vi "Calibration.vi"() -> ()   [LabVIEW 2009]
uses:
  lib/Calibration/Actuator Controls.ctl
  lib/Apps/On Off Button.ctl
  lib/Calibration/Calibration Readings.ctl
  lib/Calibration/CalibrationRampState.ctl
  lib/Calibration/SquareWaveRampState.ctl
  lib/Data Access Objects/Autobalance/Autobalance Control Parameters.ctl
  lib/Calibration/Cal Autobalance State.ctl
  lib/Apps/Yes No Button.ctl
  lib/Autobalance/Autobalance Stage.ctl
  lib/Calibration/Cal Autobalance Loop States.ctl
  lib/Autobalance/Autobalance State.ctl
  Test Utilities/DAQ Read Actions.ctl
  <vilib>/DAQmx/write.llb/DAQmx Write (Analog 1D DBL NChan 1Samp).vi
  lib/Autobalance/Autobalance Status Data.ctl
  lib/Autobalance/Autobalance Data Point.ctl
  lib/Data Access Objects/Metadata/LBCB Number.ctl
panel:
  in  "Control Type":enum32{"Set", "Ramp", "Square", "Autobalance"}(tab)=enum."Autobalance"
  in  "Set Control":cluster{"Set":bool, "Actuator Controls":T1} {"Actuator Controls"."Actuator Z2" min=-10.0 max=10.0 step=0.1 scale=-10.0..10.0; "Actuator Controls"."Actuator Z3" min=-10.0 max=10.0 step=0.1 scale=-10.0..10.0; "Actuator Controls"."Actuator X2" min=-10.0 max=10.0 step=0.1 scale=-10.0..10.0; "Actuator Controls"."Actuator Y1" min=-10.0 max=10.0 step=0.1 scale=-10.0..10.0; "Actuator Controls"."Actuator Z1" min=-10.0 max=10.0 step=0.1 scale=-10.0..10.0; "Actuator Controls"."Actuator X1" min=-10.0 max=10.0 step=0.1 scale=-10.0..10.0}
  in  "Ramp Control":T2={"Ramp Time\n(millseconds)"=30.0, "No. of Steps"=100, "Ramp"=FALSE, "Actuator Controls"={"Actuator X1"=0.0, "Actuator X2"=0.0, "Actuator Y1"=0.0, "Actuator Z1"=0.0, "Actuator Z2"=0.0, "Actuator Z3"=0.0}} {"Actuator Controls"."Actuator Z2" min=-10.0 max=10.0 step=0.1 scale=-10.0..10.0; "Actuator Controls"."Actuator Z3" min=-10.0 max=10.0 step=0.1 scale=-10.0..10.0; "Actuator Controls"."Actuator X2" min=-10.0 max=10.0 step=0.1 scale=-10.0..10.0; "Actuator Controls"."Actuator Y1" min=-10.0 max=10.0 step=0.1 scale=-10.0..10.0; "Actuator Controls"."Actuator Z1" min=-10.0 max=10.0 step=0.1 scale=-10.0..10.0; "Actuator Controls"."Actuator X1" min=-10.0 max=10.0 step=0.1 scale=-10.0..10.0}
  in  "Ramp State":T3
  in  "Square State":T4
  in  "Square Control":T5={"Hold Time\n(milliseconds)"=2000, "No. of\n Iterations"=5, "Run"=FALSE, "Actuator Controls"={"Actuator X1"=0.0, "Actuator X2"=0.0, "Actuator Y1"=0.0, "Actuator Z1"=0.0, "Actuator Z2"=0.0, "Actuator Z3"=0.0}} {"Actuator Controls"."Actuator Z2" min=-10.0 max=10.0 step=0.1 scale=-10.0..10.0; "Actuator Controls"."Actuator Z3" min=-10.0 max=10.0 step=0.1 scale=-10.0..10.0; "Actuator Controls"."Actuator X2" min=-10.0 max=10.0 step=0.1 scale=-10.0..10.0; "Actuator Controls"."Actuator Y1" min=-10.0 max=10.0 step=0.1 scale=-10.0..10.0; "Actuator Controls"."Actuator Z1" min=-10.0 max=10.0 step=0.1 scale=-10.0..10.0; "Actuator Controls"."Actuator X1" min=-10.0 max=10.0 step=0.1 scale=-10.0..10.0}
  in  "Autobalance":bool
  in  "Error Tolerance":dbl=0.005
  out "Cal Autobalance State":T6
  in  "Autobalance \nControl Parameters":T9={"Number of Samples"=30, "Delay After Cmd"=100, "Maximum Command"=9.2}
  out "Autobalance Loop State":T10 caption="State"
  out "Autobalance State Out":T11
  in  "Zoom Type":T12(ring)
  in  "Restore":bool
  in  "Zoom In":bool
  in  "Readings":T13
  in  "Actuator":i32(listbox)
  out "Readings":T14(graph)={"Average[0]"=-7.17251209904047, "Average[1]"=-8.19396103384171, "Average[2]"=-9.68369051887908, "Average[3]"=-9.45574535938537, "Average[4]"=-9.241187346298316, "Average[5]"=-8.612741694704903, "Average[6]"=0.0, "Average[7]"=0.0, "Average[8]"=0.0}
  in  "Logging":T15
  out "Command Voltage":dbl[](array[numeric])=[-0.0, -0.0, -0.0, -0.0, -0.0, -0.0]
  in  "Log File Path":path=path "C:/Documents and Settings/mbletzin/Desktop/CalVolts.txt"
  out "Control Voltage":dbl[](array[numeric])=[-0.0, -0.0, -0.0, -0.0, -0.0, -0.0]
  in  "rate":dbl=100.0
  in  "samples per channel":i32=30
  out "Servo Error Reading":dbl[](array[numeric])=[-5.882376727117365, -6.585181568259441, -9.220694636240406, -8.950128810593748, -9.598174526274564, -9.458937013781334]
  in  "Command Voltage Task":refnum<k21>="Command Voltage"
  in  "Readings Task":refnum<k21>="All Readings"
  out "Read error out":errorcluster
  out "Write error out":errorcluster
  in  "Read error in (no error)":errorcluster
  out "Load Cell \nReading":dbl[](array[numeric])=[-7.680882880270997, -8.566659800159199, -9.658116593296763, -9.594949810916727, -8.940447035067507, -8.192445315897492]
  out "LVDT Reading":dbl[](array[numeric])=[-7.17251209904047, -8.19396103384171, -9.68369051887908, -9.45574535938537, -9.241187346298316, -8.612741694704903]
  in  "Quit":bool
  # "LBCB CALIBRATION PROGRAM"
  # "Is Balanced"
  # "State"
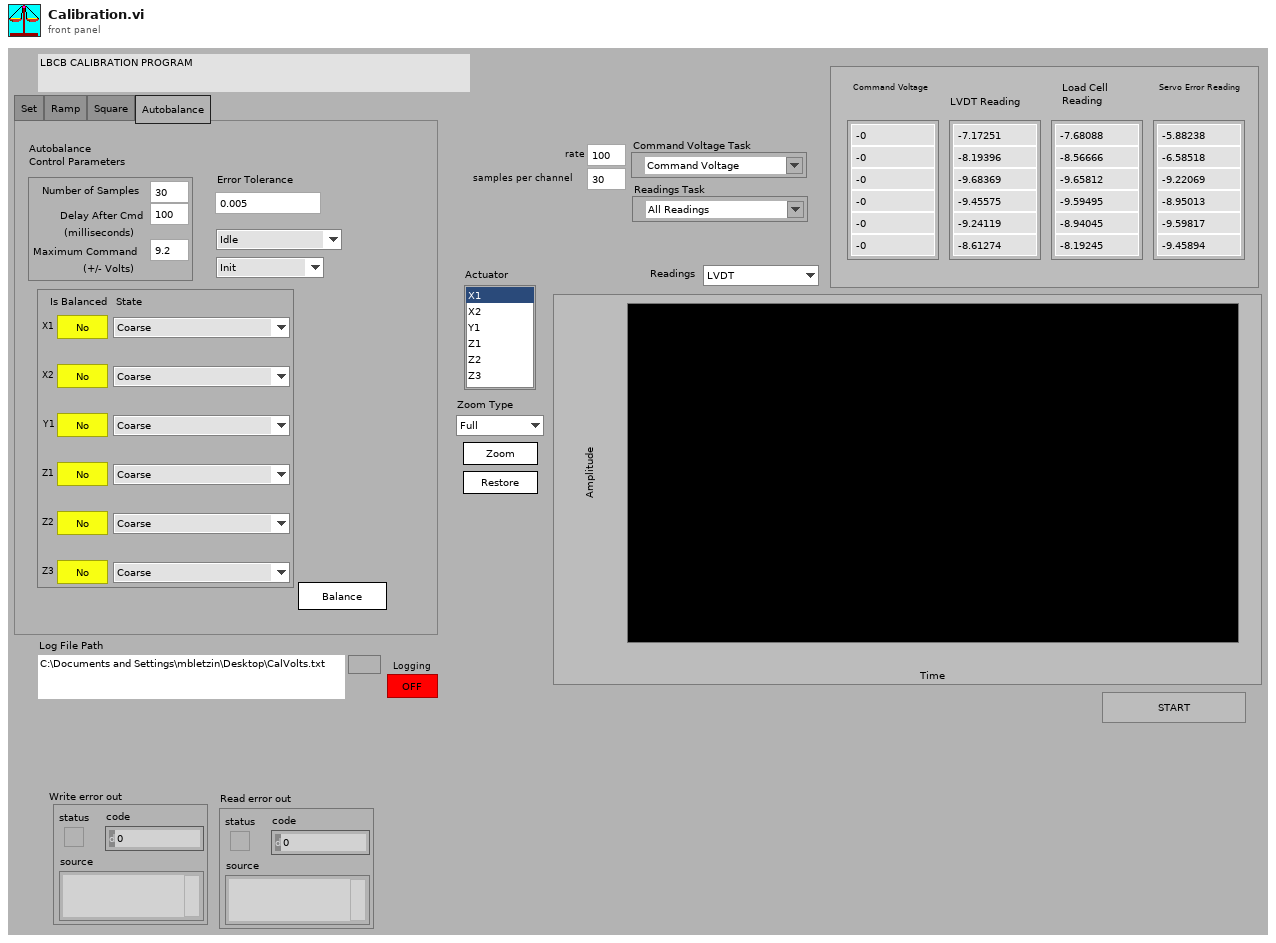
[diagram p1: front panel]
types:
  T1 = typedef "Actuator Controls.ctl" = cluster{"Actuator X1":dbl, "Actuator X2":dbl, "Actuator Y1":dbl, "Actuator Z1":dbl, "Actuator Z2":dbl, "Actuator Z3":dbl}
  T2 = cluster{"Ramp Time\n(millseconds)":dbl, "No. of Steps":i32, "Ramp":bool, "Actuator Controls":T1}
  T3 = typedef "CalibrationRampState.ctl" = enum16{"Idle", "Start Ramp", "Ramping", "Stopping"}
  T4 = typedef "SquareWaveRampState.ctl" = enum16{"Idle", "Start Wave", "High", "Low", "Stop"}
  T5 = cluster{"Hold Time\n(milliseconds)":i32, "No. of\n Iterations":i32, "Run":bool, "Actuator Controls":T1}
  T6 = typedef "Cal Autobalance State.ctl" = cluster{"X1 IsBalanced":T7, "X1 State":T8, "X2 IsBalanced":T7, "X2 State":T8, "Y1 IsBalanced":T7, "Y1 State":T8, "Z1 IsBalanced":T7, "Z1 State":T8, "Z2 IsBalanced":T7, "Z2 State":T8, "Z3 IsBalanced":T7, "Z3 State":T8}
  T7 = typedef "Yes No Button.ctl" = bool
  T8 = typedef "Autobalance Stage.ctl" = enum16{"Coarse", "Fine", "Backing Up", "Done"}
  T9 = typedef "Autobalance Control Parameters.ctl" = cluster{"Number of Samples":i32, "Delay After Cmd":i32, "Maximum Command":dbl}
  T10 = typedef "Cal Autobalance Loop States.ctl" = enum16{"Idle", "Start Balancing", "Balancing", "Stop"}
  T11 = typedef "Autobalance State.ctl" = enum16{"Init", "Send High ", "Wait High", "Read High Start", "Read High", "Send Low", "Wait Low", "Read Low Start", "Read Low", "Publish", "Calculate", "Done"}
  T12 = enum16{"Full", "Upper Half", "Upper Edge", "Lower Half", "Lower Edge"}
  T13 = typedef "Calibration Readings.ctl" = enum16{"LVDT", "Load Cell", "Servo Errors"}
  T14 = cluster{"Average[0]":dbl, "Average[1]":dbl, "Average[2]":dbl, "Average[3]":dbl, "Average[4]":dbl, "Average[5]":dbl, "Average[6]":dbl, "Average[7]":dbl, "Average[8]":dbl}
  T15 = typedef "On Off Button.ctl" = bool
  T16 = enum8{"Enabled", "Disabled", "Disabled and Grayed Out"}
  T17 = typedef "DAQ Read Actions.ctl" = enum16{"Start", "Read", "Stop"}
  T18 = typedef "Autobalance Status Data.ctl" = cluster{"IsBalanced":T7, "Autobalance Stage":T8, "High":T19, "Low":T19, "Balanced \nCmd":dbl}
  T19 = typedef "Autobalance Data Point.ctl" = cluster{"cCmd":dbl, "cServo":dbl, "pCmd":dbl, "pServo":dbl}
  T20 = typedef "LBCB Number.ctl" = enum16{"LBCB1", "LBCB2"}
  T21 = cluster{"Average[0]":dbl, "Average[1]":dbl, "Average[2]":dbl, "Average[3]":dbl, "Average[4]":dbl, "Average[5]":dbl, "Average[6]":dbl, "Average[7]":dbl, "Average[8]":dbl}[]
  T22 = enum16{"open", "replace", "create", "open or create", "replace or create", "replace or create with confirmation"}
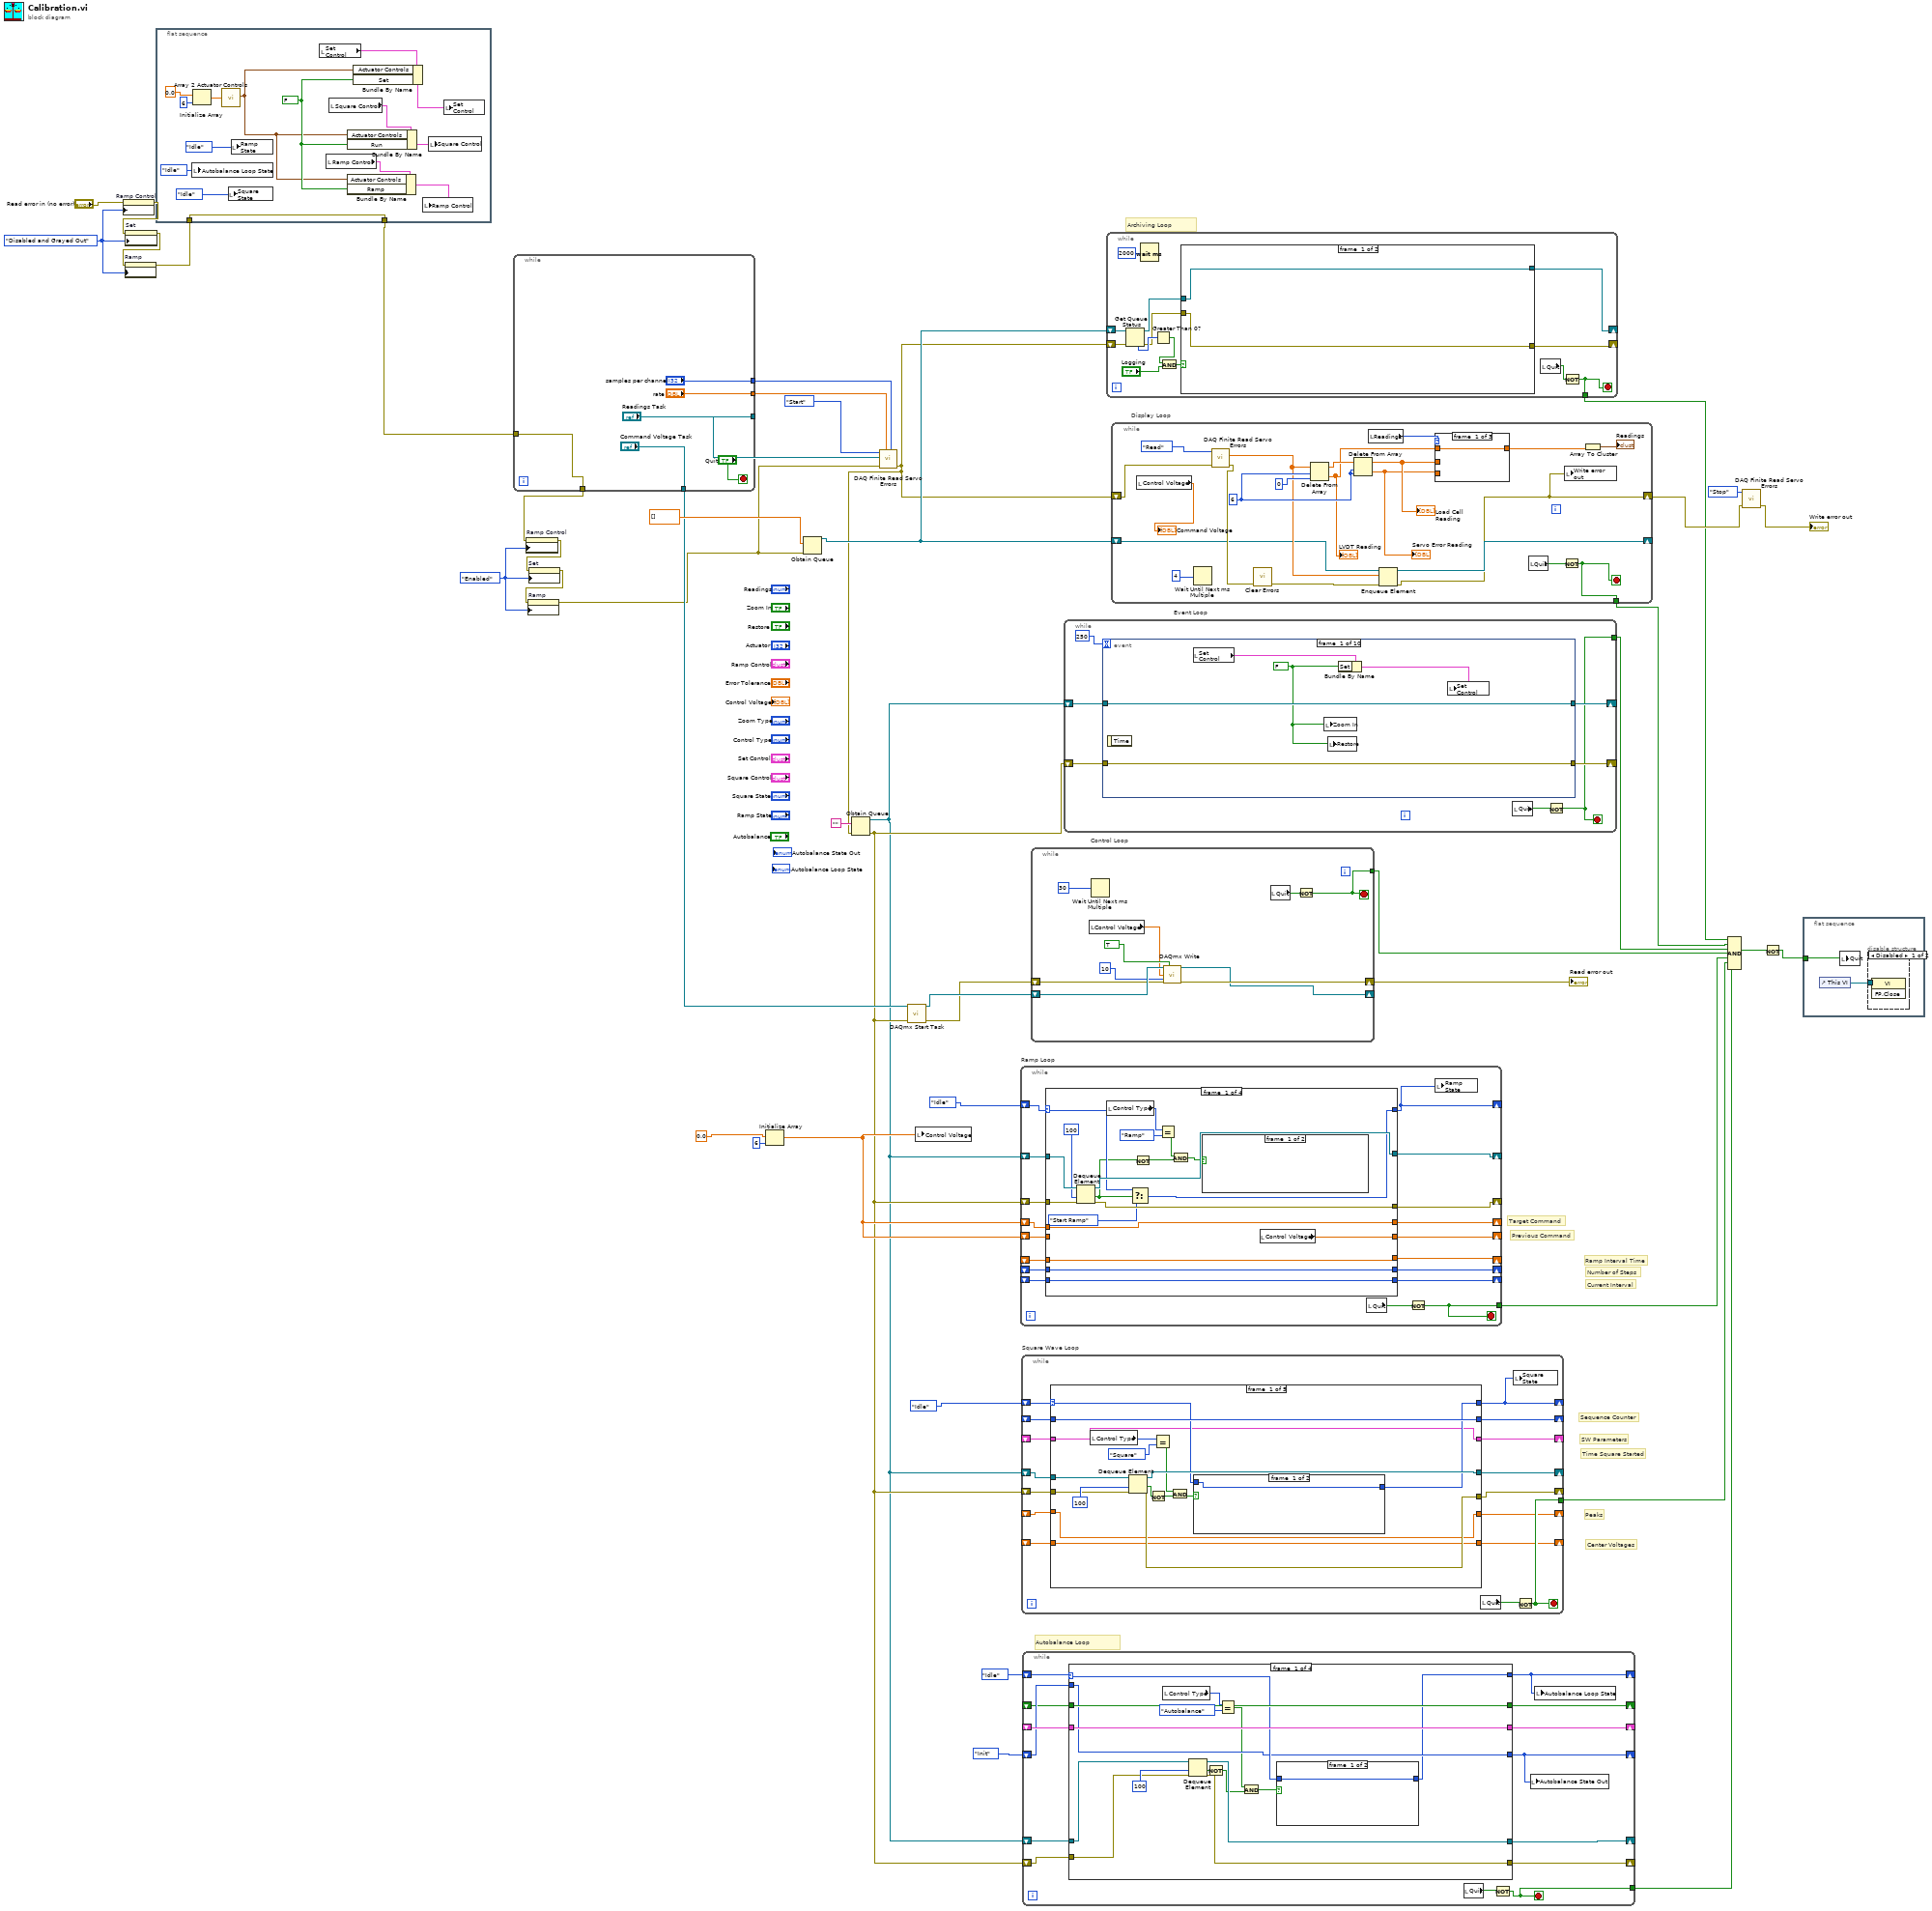
[diagram p0: block diagram]
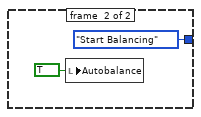
[diagram p2: hidden frame]
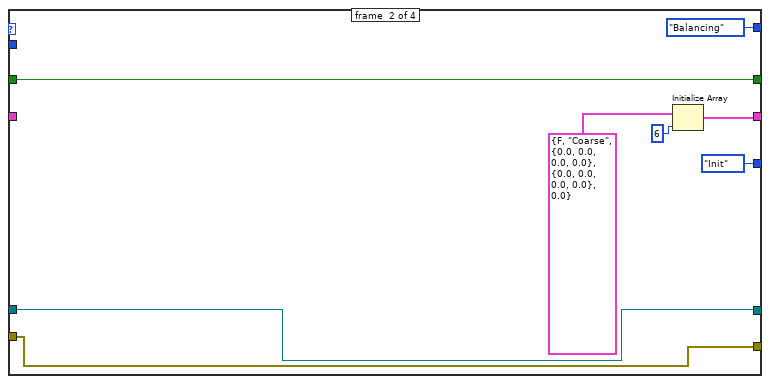
[diagram p3: hidden frame]
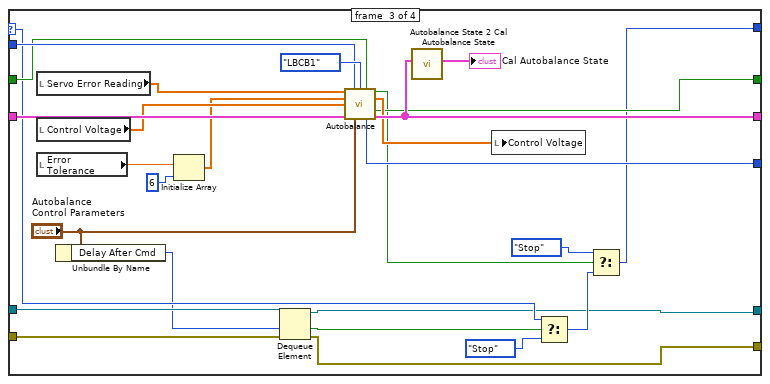
[diagram p4: hidden frame]
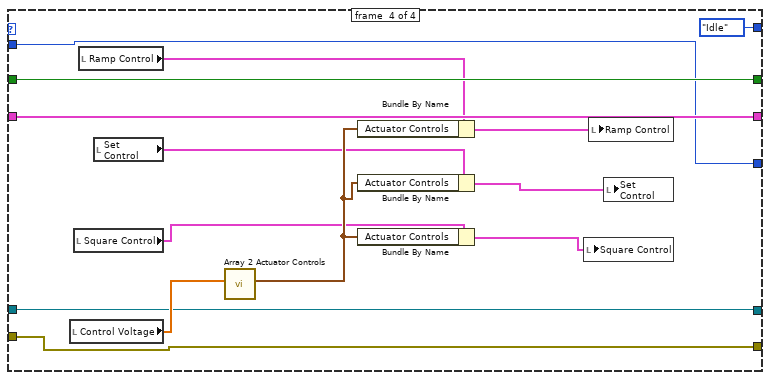
[diagram p5: hidden frame]
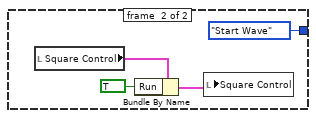
[diagram p6: hidden frame]
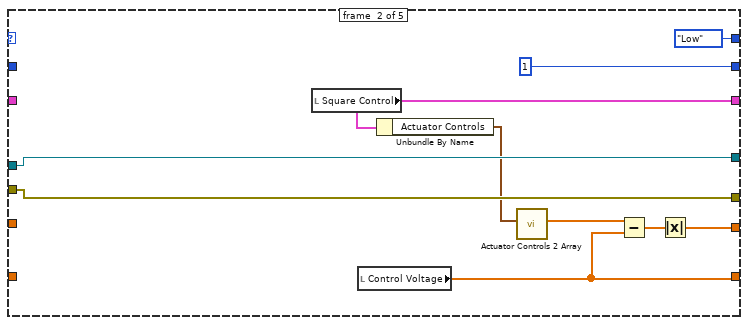
[diagram p7: hidden frame]
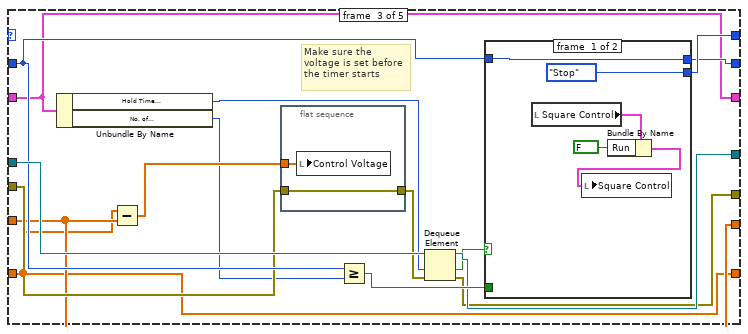
[diagram p8: hidden frame]
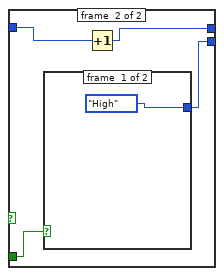
[diagram p9: hidden frame]
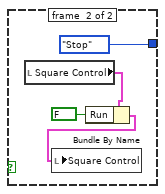
[diagram p10: hidden frame]
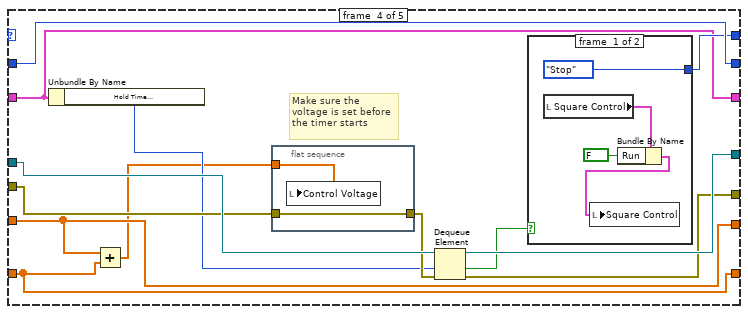
[diagram p11: hidden frame]
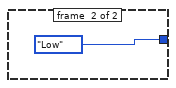
[diagram p12: hidden frame]
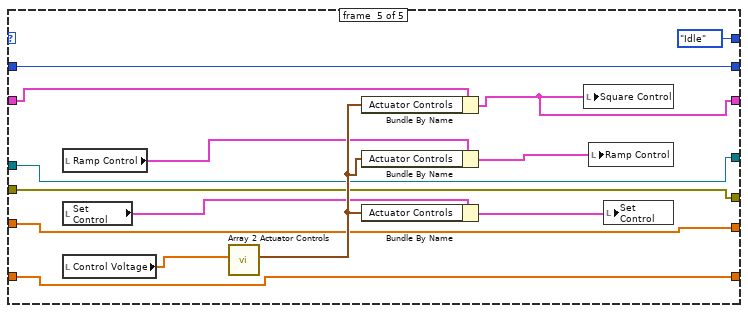
[diagram p13: hidden frame]
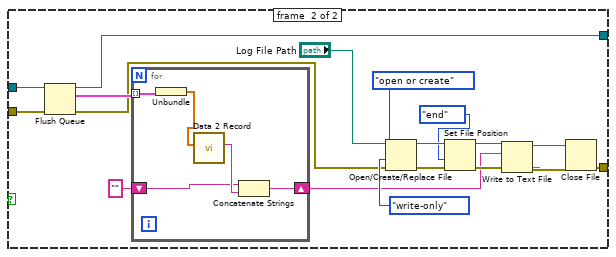
[diagram p15: hidden frame]
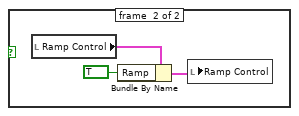
[diagram p16: hidden frame]
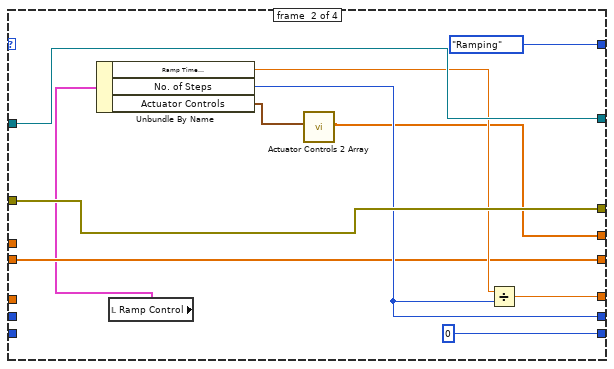
[diagram p17: hidden frame]
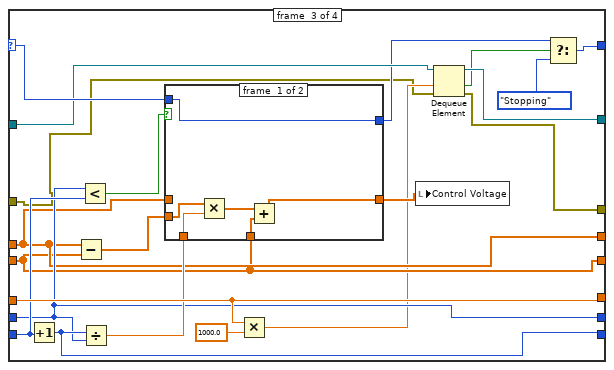
[diagram p18: hidden frame]
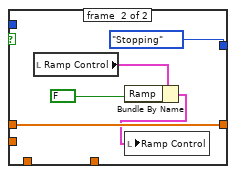
[diagram p19: hidden frame]
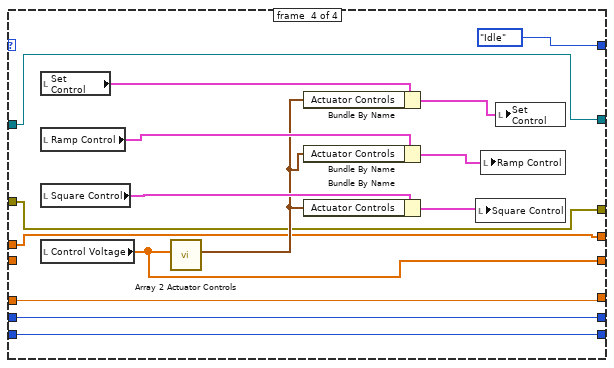
[diagram p20: hidden frame]
diagram:
  w13 = T16."Enabled" ("Disabled")
  w16 = T16."Disabled and Grayed Out" ("Disabled")
  # "Autobalance Loop"
  # "Peaks"
  # "Center Voltages"
  # "Archiving Loop"
  # "Time Square Started"
  # "SW Parameters"
  # "Sequence Counter"
  # "Previous Command"
  # "Target Command"
  # "Ramp Interval Time"
  # "Number of Steps"
  # "Current Interval"
  n1 = property on="Ramp Control" class="Clust (strict)"(error in="Read error in (no error)", "DisabledEnum"=w16) -> (error out=w18:errorcluster)  [unwired: 1 in, 1 out]
  n2 = property on="Set" class="Bool (strict)"(error in=w18, "DisabledEnum"=w16) -> (error out=w17:errorcluster)  [unwired: 1 in, 1 out]
  n3 = property on="Ramp" class="Bool (strict)"(error in=w17, "DisabledEnum"=w16) -> (error out=w2:errorcluster)  [unwired: 1 in, 1 out]
  n4 = flat-sequence {
    tunnel: w2 -> [w48]
    tunnel: [w48] -> w1
    frame #0 {
      w56 = FALSE
      n5 = local write "Autobalance Loop State"(Cal_Autobalance_Loop_States."Idle" ("Autobalance Loop State")) -> ()
      n6 = Initialize Array(0.0 ("element"), 6 ("dimension size")) -> (w57:dbl[])
      n7 = call "Array 2 Actuator Controls.vi"("Array"=w57) -> ("Actuator Controls"=w49:T1)  [unwired: 10 in]
      n8 = local write "Square State"(SquareWaveRampState."Idle" ("Square State")) -> ()
      n9 = local write "Ramp State"(CalibrationRampState."Idle" ("Ramp State")) -> ()
      n10 = local read "Set Control"() -> (w52:cluster{"Set":bool, "Actuator Controls":T1})
      n11 = local read "Ramp Control"() -> (w50:T2)
      n12 = local read "Square Control"() -> (w54:T5)
      n13 = Bundle By Name(cluster=w50, "Actuator Controls"=w49, "Ramp"=w56) -> (w51:T2)
      n14 = Bundle By Name(cluster=w54, "Actuator Controls"=w49, "Run"=w56) -> (w55:T5)
      n15 = Bundle By Name(cluster=w52, "Actuator Controls"=w49, "Set"=w56) -> (w53:cluster{"Set":bool, "Actuator Controls":T1})
      n16 = local write "Ramp Control"(w51) -> ()
      n17 = local write "Square Control"(w55) -> ()
      n18 = local write "Set Control"(w53) -> ()
    }
  }
  n19 = while {
    tunnel: [w60] -> w12
    tunnel: ["samples per channel"] -> w25
    tunnel: ["rate"] -> w24
    tunnel: ["Readings Task"] -> w23
    tunnel: ["Command Voltage Task"] -> w21
    tunnel: w1 -> [w60]
    stop <- "Quit" stop-if-true
  }
  n20 = property on="Ramp Control" class="Clust (strict)"(error in=w12, "DisabledEnum"=w13) -> (error out=w15:errorcluster)  [unwired: 1 in, 1 out]
  n21 = property on="Set" class="Bool (strict)"(error in=w15, "DisabledEnum"=w13) -> (error out=w14:errorcluster)  [unwired: 1 in, 1 out]
  n22 = property on="Ramp" class="Bool (strict)"(error in=w14, "DisabledEnum"=w13) -> (error out=w11:errorcluster)  [unwired: 1 in, 1 out]
  n23 = Initialize Array(0.0 ("element"), 6 ("dimension size")) -> (w20:dbl[])
  n24 = Obtain Queue(element data type=dbl[] [], error in (no error)=w11) -> (queue out=w29:refnum<queue>)  [unwired: 3 in, 2 out]
  n25 = call "DAQ Finite Read Servo Errors.vi"("samples per channel"=w25, "rate"=w24, "error in"=w11, "task/channels in"=w23, "Action"=DAQ_Read_Actions."Start") -> ("error out"=w22:errorcluster)  [unwired: 6 out]
  n26 = Obtain Queue(element data type="", error in (no error)=w22) -> (queue out=w3:refnum<queue>, error out=w4:errorcluster)  [unwired: 3 in, 1 out]
  n27 = call <vilib>:"DAQmx Start Task.vi"("task/channels in"=w21, "error in"=w4) -> ("task out"=w44:refnum<k21>, "error out"=w8:errorcluster)  [unwired: 12 out]
  n28 = local write "Control Voltage"(w20) -> ()
  n29 = while "Ramp Loop" {
    shift-right: [w66] -> _
    shift-left: CalibrationRampState."Idle" ("Ramp State") -> [w83]
    shift-right: [w80] -> _
    shift-left: w3 -> [w82]
    shift-right: [w79] -> _
    shift-left: w4 -> [w81]
    shift-right: [w78] -> _
    shift-left: _ -> [w70]
    shift-right: [w76] -> _
    shift-left: _ -> [w71]
    shift-right: [w77] -> _
    shift-left: _ -> [w72]
    shift-right: [w75] -> _
    shift-left: w20 -> [w73]
    shift-right: [w74] -> _
    shift-left: w20 -> [w69]
    tunnel: [w67] -> w31
    stop <- w67 stop-if-true
    n30 = case shown="\"Idle\"" w83 {
      selector: w83 -> [w97 _ w128 _]
      tunnel: w82 -> [w102 w115 w127 w154]
      tunnel: w81 -> [w101 w116 w119 w149]
      tunnel: [w99 w115 w124 w154] -> w80
      tunnel: [w98 w116 w118 w149] -> w79
      tunnel: [w96 CalibrationRampState."Ramping" ("f") w121 CalibrationRampState."Idle" ("f")] -> w66
      tunnel: [w92 w112 w136 w152] -> w78
      tunnel: [w90 0 w135 w150] -> w77
      tunnel: [w91 w110 w129 w151] -> w76
      tunnel: [w94 w109 w125 w155] -> w75
      tunnel: [w93 w106 w126 w156] -> w74
      tunnel: w73 -> [_ w109 w125 _]
      tunnel: w72 -> [w90 _ w130 w150]
      tunnel: w71 -> [w91 _ w129 w151]
      tunnel: w70 -> [w92 _ w136 w152]
      tunnel: w69 -> [w93 _ w126 w156]
      frame #0 {
        n31 = Dequeue Element(queue=w102, timeout in ms (-1)=100, error in (no error)=w101) -> (queue out=w99:refnum<queue>, timed out?=w89:bool, error out=w98:errorcluster)  [unwired: 1 out]
        n32 = local read "Control Type"() -> (w88:enum32{"Set", "Ramp", "Square", "Autobalance"})
        n33 = Select(t=w97, s=w89, f=CalibrationRampState."Start Ramp") -> (s? t:f=w96:T3)
        n34 = Not(x=w89) -> (.not. x?=w84:bool)
        n35 = Equal?(x=w88, y=enum32{"Set", "Ramp", "Square", "Autobalance"}."Ramp") -> (x = y?=w86:bool)
        n36 = And(x=w86, y=w84) -> (x .and. y?=w87:bool)
        n37 = case shown="False" w87 {
          frame #0 {
          }
          frame #1 {
            n38 = local read "Ramp Control"() -> (w105:T2)
            n39 = Bundle By Name(cluster=w105, "Ramp"=TRUE) -> (w104:T2)
            n40 = local write "Ramp Control"(w104) -> ()
          }
        }
        n41 = local read "Control Voltage"() -> (w94:dbl[])
      }
      frame #1 {
        n42 = local read "Ramp Control"() -> (w108:T2)
        n43 = Unbundle By Name(w108) -> ("Ramp Time\n(millseconds)"=w113:dbl, "No. of Steps"=w110:i32, "Actuator Controls"=w107:T1)
        n44 = call "Actuator Controls 2 Array.vi"("Actuator Controls"=w107) -> ("Array"=w106:dbl[])  [unwired: 10 in]
        n45 = Divide(x=w113, y=w110) -> (x/y=w112:dbl)
      }
      frame #2 {
        n46 = Increment(x=w130) -> (x+1=w135:i32)
        n47 = Subtract(x=w126, y=w125) -> (x-y=w134:dbl[])
        n48 = Less?(x=w129, y=w130) -> (x < y?=w131:bool)
        n49 = Divide(x=w135, y=w129) -> (x/y=w133:dbl)
        n50 = case shown="False" w131 {
          tunnel: w134 -> [w143 _]
          tunnel: w133 -> [w142 _]
          tunnel: [w139 w147] -> w132
          tunnel: w128 -> [w140 _]
          tunnel: [w140 CalibrationRampState."Stopping" ("Ramp State")] -> w122
          tunnel: w126 -> [_ w147]
          tunnel: w125 -> [w138 _]
          frame #0 {
            n51 = Multiply(x=w143, y=w142) -> (x*y=w141:dbl[])
            n52 = Add(x=w141, y=w138) -> (x+y=w139:dbl[])
          }
          frame #1 {
            n53 = local read "Ramp Control"() -> (w146:T2)
            n54 = Bundle By Name(cluster=w146, "Ramp"=FALSE) -> (w145:T2)
            n55 = local write "Ramp Control"(w145) -> ()
          }
        }
        n56 = Multiply(x=w136, y=1000.0) -> (x*y=w123:dbl)
        n57 = local write "Control Voltage"(w132) -> ()
        n58 = Dequeue Element(queue=w127, timeout in ms (-1)=w123, error in (no error)=w119) -> (queue out=w124:refnum<queue>, timed out?=w117:bool, error out=w118:errorcluster)  [unwired: 1 out]
        n59 = Select(t=w122, s=w117, f=CalibrationRampState."Stopping") -> (s? t:f=w121:T3)
      }
      frame #3 {
        n60 = local read "Set Control"() -> (w163:cluster{"Set":bool, "Actuator Controls":T1})
        n61 = local read "Ramp Control"() -> (w162:T2)
        n62 = local read "Square Control"() -> (w161:T5)
        n63 = local read "Control Voltage"() -> (w155:dbl[])
        n64 = call "Array 2 Actuator Controls.vi"("Array"=w155) -> ("Actuator Controls"=w160:T1)  [unwired: 10 in]
        n65 = Bundle By Name(cluster=w163, "Actuator Controls"=w160) -> (w159:cluster{"Set":bool, "Actuator Controls":T1})
        n66 = Bundle By Name(cluster=w162, "Actuator Controls"=w160) -> (w158:T2)
        n67 = Bundle By Name(cluster=w161, "Actuator Controls"=w160) -> (w157:T5)
        n68 = local write "Square Control"(w157) -> ()
        n69 = local write "Ramp Control"(w158) -> ()
        n70 = local write "Set Control"(w159) -> ()
      }
    }
    n71 = local read "Quit"() -> (w68:bool)
    n72 = Not(x=w68) -> (.not. x?=w67:bool)
    n73 = local write "Ramp State"(w66) -> ()
  }
  n74 = while "Square Wave Loop" {
    tunnel: [w177] -> w9
    shift-right: [w175] -> _
    shift-left: w4 -> [w176]
    shift-right: [w173] -> _
    shift-left: w3 -> [w174]
    shift-right: [w172] -> _
    shift-left: SquareWaveRampState."Idle" ("Square State") -> [w179]
    shift-right: [w171] -> _
    shift-left: _ -> [w170]
    shift-right: [w169] -> _
    shift-left: _ -> [w167]
    shift-right: [w168] -> _
    shift-left: _ -> [w166]
    shift-right: [w165] -> _
    shift-left: _ -> [w164]
    stop <- w177 stop-if-true
    n75 = case shown="\"Idle\"" w179 {
      selector: w179 -> [w191 _ _ _ _]
      tunnel: w176 -> [w195 w211 w219 w254 w266]
      tunnel: [w189 w211 w221 w250 w266] -> w175
      tunnel: w174 -> [w194 w210 w224 w256 w267]
      tunnel: [w193 w210 w222 w255 w267] -> w173
      tunnel: [w190 SquareWaveRampState."Low" ("Square State") w227 w248 SquareWaveRampState."Idle" ("t")] -> w172
      tunnel: [w192 1 w225 w251 w269] -> w171
      tunnel: w170 -> [w192 _ w223 w251 w269]
      tunnel: [w187 w205 w212 w247 w264] -> w169
      tunnel: [w188 w203 w213 w246 w265] -> w168
      tunnel: w167 -> [w187 _ w212 w247 w264]
      tunnel: w166 -> [w188 _ w213 w246 w265]
      tunnel: [w186 w202 w214 w244 w268] -> w165
      tunnel: w164 -> [w186 _ w214 w244 w275]
      frame #0 {
        n76 = local read "Control Type"() -> (w181:enum32{"Set", "Ramp", "Square", "Autobalance"})
        n77 = Dequeue Element(queue=w194, timeout in ms (-1)=100, error in (no error)=w195) -> (queue out=w193:refnum<queue>, timed out?=w184:bool, error out=w189:errorcluster)  [unwired: 1 out]
        n78 = Not(x=w184) -> (.not. x?=w180:bool)
        n79 = Equal?(x=w181, y=enum32{"Set", "Ramp", "Square", "Autobalance"}."Square") -> (x = y?=w185:bool)
        n80 = And(x=w185, y=w180) -> (x .and. y?=w183:bool)
        n81 = case shown="False" w183 {
          tunnel: w191 -> [w197 _]
          tunnel: [w197 SquareWaveRampState."Start Wave" ("Square State")] -> w190
          frame #0 {
          }
          frame #1 {
            n82 = local read "Square Control"() -> (w201:T5)
            n83 = Bundle By Name(cluster=w201, "Run"=TRUE) -> (w200:T5)
            n84 = local write "Square Control"(w200) -> ()
          }
        }
      }
      frame #1 {
        n85 = local read "Square Control"() -> (w202:T5)
        n86 = local read "Control Voltage"() -> (w205:dbl[])
        n87 = Unbundle By Name(w202) -> ("Actuator Controls"=w207:T1)
        n88 = call "Actuator Controls 2 Array.vi"("Actuator Controls"=w207) -> ("Array"=w206:dbl[])  [unwired: 10 in]
        n89 = Subtract(x=w206, y=w205) -> (x-y=w204:dbl[])
        n90 = Absolute Value(x=w204) -> (abs(x)=w203:dbl[])
      }
      frame #2 {
        # "Make sure the \nvoltage is set before\nthe timer starts"
        n91 = Unbundle By Name(w214) -> ("Hold Time\n(milliseconds)"=w215:i32, "No. of\n Iterations"=w216:i32)
        n92 = Subtract(x=w212, y=w213) -> (x-y=w217:dbl[])
        n93 = flat-sequence {
          tunnel: w219 -> [w229]
          tunnel: [w229] -> w218
          tunnel: w217 -> [w228]
          frame #0 {
            n94 = local write "Control Voltage"(w228) -> ()
          }
        }
        n95 = Greater Or Equal?(x=w223, y=w216) -> (x >= y?=w226:bool)
        n96 = Dequeue Element(queue=w224, timeout in ms (-1)=w215, error in (no error)=w218) -> (queue out=w222:refnum<queue>, timed out?=w220:bool, error out=w221:errorcluster)  [unwired: 1 out]
        n97 = case shown="False" w220 {
          tunnel: [SquareWaveRampState."Stop" ("t") w235] -> w227
          tunnel: w226 -> [_ w236]
          tunnel: w223 -> [w234 w238]
          tunnel: [w234 w237] -> w225
          frame #0 {
            n98 = local read "Square Control"() -> (w232:T5)
            n99 = Bundle By Name(cluster=w232, "Run"=FALSE) -> (w231:T5)
            n100 = local write "Square Control"(w231) -> ()
          }
          frame #1 {
            n101 = case shown="True" w236 {
              tunnel: [SquareWaveRampState."High" ("t") SquareWaveRampState."Stop" ("t")] -> w235
              frame #0 {
              }
              frame #1 {
                n102 = local read "Square Control"() -> (w242:T5)
                n103 = Bundle By Name(cluster=w242, "Run"=FALSE) -> (w240:T5)
                n104 = local write "Square Control"(w240) -> ()
              }
            }
            n105 = Increment(x=w238) -> (x+1=w237:i32)
          }
        }
      }
      frame #3 {
        # "Make sure the \nvoltage is set before\nthe timer starts"
        n106 = Unbundle By Name(w244) -> ("Hold Time\n(milliseconds)"=w252:i32)
        n107 = Add(x=w246, y=w247) -> (x+y=w245:dbl[])
        n108 = flat-sequence {
          tunnel: w254 -> [w263]
          tunnel: [w263] -> w253
          tunnel: w245 -> [w262]
          frame #0 {
            n109 = local write "Control Voltage"(w262) -> ()
          }
        }
        n110 = Dequeue Element(queue=w256, timeout in ms (-1)=w252, error in (no error)=w253) -> (queue out=w255:refnum<queue>, timed out?=w249:bool, error out=w250:errorcluster)  [unwired: 1 out]
        n111 = case shown="False" w249 {
          tunnel: [SquareWaveRampState."Stop" ("t") SquareWaveRampState."Low" ("t")] -> w248
          frame #0 {
            n112 = local read "Square Control"() -> (w259:T5)
            n113 = Bundle By Name(cluster=w259, "Run"=FALSE) -> (w257:T5)
            n114 = local write "Square Control"(w257) -> ()
          }
          frame #1 {
          }
        }
      }
      frame #4 {
        n115 = local read "Ramp Control"() -> (w274:T2)
        n116 = local read "Set Control"() -> (w272:cluster{"Set":bool, "Actuator Controls":T1})
        n117 = local read "Control Voltage"() -> (w276:dbl[])
        n118 = call "Array 2 Actuator Controls.vi"("Array"=w276) -> ("Actuator Controls"=w277:T1)  [unwired: 10 in]
        n119 = Bundle By Name(cluster=w275, "Actuator Controls"=w277) -> (w268:T5)
        n120 = Bundle By Name(cluster=w274, "Actuator Controls"=w277) -> (w273:T2)
        n121 = Bundle By Name(cluster=w272, "Actuator Controls"=w277) -> (w271:cluster{"Set":bool, "Actuator Controls":T1})
        n122 = local write "Square Control"(w268) -> ()
        n123 = local write "Ramp Control"(w273) -> ()
        n124 = local write "Set Control"(w271) -> ()
      }
    }
    n125 = local read "Quit"() -> (w178:bool)
    n126 = local write "Square State"(w172) -> ()
    n127 = Not(x=w178) -> (.not. x?=w177:bool)
  }
  n128 = while {
    shift-right: [w278] -> _
    shift-left: Cal_Autobalance_Loop_States."Idle" ("Square State") -> [w291]
    shift-right: [w289] -> _
    shift-left: _ -> [w290]
    shift-right: [w279] -> _
    shift-left: Autobalance_State."Init" ("Autobalance State Out") -> [w288]
    shift-right: [w287] -> _
    shift-left: _ -> [w286]
    shift-right: [w281] -> _
    shift-left: w4 -> [w283]
    shift-right: [w282] -> _
    shift-left: w3 -> [w284]
    tunnel: [w280] -> w5
    stop <- w280 stop-if-true
    n129 = case shown="\"Idle\"" w291 {
      selector: w291 -> [w299 _ w325 _]
      tunnel: w290 -> [w306 _ w344 w357]
      tunnel: [w306 w316 w342 w357] -> w289
      tunnel: [w298 Autobalance_State."Init" ("Autobalance State Out") w340 w356] -> w279
      tunnel: w288 -> [w298 _ w339 w356]
      tunnel: [w307 w314 w333 w358] -> w287
      tunnel: w286 -> [w307 w314 w332 w358]
      tunnel: [w297 Cal_Autobalance_Loop_States."Balancing" ("Square State") w329 Cal_Autobalance_Loop_States."Idle" ("Square State")] -> w278
      tunnel: w284 -> [w304 w312 w324 w347]
      tunnel: w283 -> [w302 w311 w323 w346]
      tunnel: [w303 w312 w322 w347] -> w282
      tunnel: [w301 w311 w321 w346] -> w281
      frame #0 {
        n130 = local read "Control Type"() -> (w293:enum32{"Set", "Ramp", "Square", "Autobalance"})
        n131 = Dequeue Element(queue=w304, timeout in ms (-1)=100, error in (no error)=w302) -> (queue out=w303:refnum<queue>, timed out?=w300:bool, error out=w301:errorcluster)  [unwired: 1 out]
        n132 = Not(x=w300) -> (.not. x?=w295:bool)
        n133 = Equal?(x=w293, y=enum32{"Set", "Ramp", "Square", "Autobalance"}."Autobalance") -> (x = y?=w296:bool)
        n134 = And(x=w296, y=w295) -> (x .and. y?=w294:bool)
        n135 = case shown="False" w294 {
          tunnel: w299 -> [w308 _]
          tunnel: [w308 Cal_Autobalance_Loop_States."Start Balancing" ("Square State")] -> w297
          frame #0 {
          }
          frame #1 {
            n136 = local write "Autobalance"(TRUE ("Autobalance")) -> ()
          }
        }
      }
      frame #1 {
        n137 = Initialize Array(T18 {"IsBalanced"=FALSE, "Autobalance Stage"=enum."Coarse", "High"={"cCmd"=0.0, "cServo"=0.0, "pCmd"=0.0, "pServo"=0.0}, "Low"={"cCmd"=0.0, "cServo"=0.0, "pCmd"=0.0, "pServo"=0.0}, "Balanced \nCmd"=0.0} ("Autobalance Persistant Values Out"), 6 ("dimension size")) -> (w316:T18[])
      }
      frame #2 {
        n138 = local read "Servo Error Reading"() -> (w345:dbl[])
        n139 = local read "Control Voltage"() -> (w338:dbl[])
        n140 = local read "Error Tolerance"() -> (w337:dbl)
        n141 = Unbundle By Name("Autobalance \nControl Parameters") -> ("Delay After Cmd"=w319:i32)
        n142 = Initialize Array(w337, 6 ("dimension size")) -> (w336:dbl[])
        n143 = Dequeue Element(queue=w324, timeout in ms (-1)=w319, error in (no error)=w323) -> (queue out=w322:refnum<queue>, timed out?=w328:bool, error out=w321:errorcluster)  [unwired: 1 out]
        n144 = call "Autobalance.vi"("Servo Errors"=w345, 1:"Autobalance State In"=w339, "LBCB Number"=LBCB_Number."LBCB1", "InitialPosition? In"=w332, "Error Tolerance"=w336, "Command In"=w338, 11:"Autobalance State In"=w344, "Autobalance \nControl Parameters"="Autobalance \nControl Parameters") -> ("IsBalanced"=w330:T7, "Command Out"=w334:dbl[], "InitialPosition? Out"=w333:T7, 14:"Autobalance State Out"=w340:T11, 15:"Autobalance State Out"=w342:T18[])  [unwired: 3 in]
        n145 = call "Autobalance State 2 Cal Autobalance State.vi"("Autobalance State In"=w342) -> ("Cal Autobalance State"=→"Cal Autobalance State":T6)  [unwired: 10 in]
        n146 = local write "Control Voltage"(w334) -> ()
        n147 = Select(t=w325, s=w328, f=Cal_Autobalance_Loop_States."Stop" ("Square State")) -> (s? t:f=w326:T10)
        n148 = Select(t=Cal_Autobalance_Loop_States."Stop" ("Square State"), s=w330, f=w326) -> (s? t:f=w329:T10)
      }
      frame #3 {
        n149 = local read "Control Voltage"() -> (w351:dbl[])
        n150 = local read "Square Control"() -> (w352:T5)
        n151 = local read "Ramp Control"() -> (w354:T2)
        n152 = local read "Set Control"() -> (w353:cluster{"Set":bool, "Actuator Controls":T1})
        n153 = call "Array 2 Actuator Controls.vi"("Array"=w351) -> ("Actuator Controls"=w355:T1)  [unwired: 10 in]
        n154 = Bundle By Name(cluster=w354, "Actuator Controls"=w355) -> (w348:T2)
        n155 = Bundle By Name(cluster=w353, "Actuator Controls"=w355) -> (w349:cluster{"Set":bool, "Actuator Controls":T1})
        n156 = Bundle By Name(cluster=w352, "Actuator Controls"=w355) -> (w350:T5)
        n157 = local write "Square Control"(w350) -> ()
        n158 = local write "Ramp Control"(w348) -> ()
        n159 = local write "Set Control"(w349) -> ()
      }
    }
    n160 = local read "Quit"() -> (w285:bool)
    n161 = Not(x=w285) -> (.not. x?=w280:bool)
    n162 = local write "Autobalance State Out"(w279) -> ()
    n163 = local write "Autobalance Loop State"(w278) -> ()
  }
  n164 = while "Control Loop" {
    shift-right: [w366] -> _
    shift-left: w44 -> [w369]
    shift-right: [w367] -> w43
    shift-left: w8 -> [w368]
    tunnel: [w360] -> w38
    stop <- w360 stop-if-true
    n165 = local read "Control Voltage"() -> (w361:dbl[])
    n166 = Wait Until Next ms Multiple(millisecond multiple=30) -> ()  [unwired: 1 out]
    n167 = call-poly <vilib>:"DAQmx Write.vi"("task/channels in"=w369, "auto start"=TRUE, "data"=w361, "timeout"=10, "error in"=w368) -> ("task out"=w366:refnum<k21>, "error out"=w367:errorcluster)  [unwired: 9 out]
    n168 = local read "Quit"() -> (w362:bool)
    n169 = Not(x=w362) -> (.not. x?=w360:bool)
  }
  "Read error out" <- w43
  n170 = while "Event Loop" {
    tunnel: [w370] -> w42
    shift-right: [w371] -> _
    shift-left: w4 -> [w373]
    shift-right: [w372] -> _
    shift-left: w3 -> [w374]
    stop <- w370 stop-if-true
    n171 = event shown="[5] \"Set Control.Set\": Mouse Down" {
      selector: _ -> [_ _ _ _ _ _ _ _ _ _]
      dyn-events: _ -> [_ _ _ _ _ _ _ _ _ _]
      timeout: 250 -> [_ _ _ _ _ _ _ _ _ _]
      tunnel: w374 -> [w381 w387 w409 w421 w440 w471 w476 w478 w505 w546]
      tunnel: w373 -> [w380 w386 w408 w420 w443 w472 w475 w483 w504 w548]
      tunnel: [w381 w385 w407 w419 w439 w471 w476 w478 w505 w546] -> w372
      tunnel: [w380 w384 w406 w418 w442 w472 w475 w479 w501 w547] -> w371
      event #0 {
        w379 = FALSE ("Set")
        n172 = event-data() -> ()  [unwired: 2 out]
        n173 = local read "Set Control"() -> (w377:cluster{"Set":bool, "Actuator Controls":T1})
        n174 = local write "Zoom In"(w379) -> ()
        n175 = local write "Restore"(w379) -> ()
        n176 = Bundle By Name(cluster=w377, "Set"=w379) -> (w378:cluster{"Set":bool, "Actuator Controls":T1})
        n177 = local write "Set Control"(w378) -> ()
      }
      event #1 {
        n178 = event-data() -> ()  [unwired: 2 out]
        n179 = local read "Ramp State"() -> (w383:T3)
        n180 = case shown="\"Stopping\"" w383 {
          tunnel: w387 -> [w392 w397 w400 w403]
          tunnel: w386 -> [w390 w395 w399 w402]
          tunnel: [w389 w394 w400 w403] -> w385
          tunnel: [w388 w393 w399 w402] -> w384
          tunnel: [_ _ TRUE TRUE] -> w382
          frame #0 {
            n181 = Enqueue Element(queue=w392, element="Start" ("notification"), error in (no error)=w390) -> (queue out=w389:refnum<queue>, error out=w388:errorcluster)  [unwired: 1 in, 1 out]
          }
          frame #1 {
            n182 = Enqueue Element(queue=w397, element="Stop" ("notification"), error in (no error)=w395) -> (queue out=w394:refnum<queue>, error out=w393:errorcluster)  [unwired: 1 in, 1 out]
          }
          frame #2 {
          }
          frame #3 {
          }
        }
        n183 = event-data("Discard?"=w382) -> ()  [unwired: 1 in, 1 out]
      }
      event #2 {
        n184 = event-data() -> ("Button"=w405:u16)  [unwired: 1 out]
        n185 = flat-sequence {
          tunnel: w409 -> [w415]
          tunnel: w408 -> [w414]
          tunnel: [w413] -> w407
          tunnel: [w412] -> w406
          tunnel: w405 -> [w411]
          tunnel: [w411] -> w404
          frame #0 {
            n186 = Flush Queue(queue=w415, error in (no error)=w414) -> (queue out=w413:refnum<queue>, error out=w412:errorcluster)  [unwired: 1 out]
          }
        }
        n187 = event-data("Button"=w404, "Discard?"=FALSE) -> ()  [unwired: 1 in, 1 out]
      }
      event #3 {
        n188 = event-data() -> ()  [unwired: 2 out]
        n189 = local read "Autobalance Loop State"() -> (w417:T10)
        n190 = case shown="\"Balancing\"" w417 {
          tunnel: w421 -> [w426 w429 w434 w437]
          tunnel: w420 -> [w424 w428 w432 w436]
          tunnel: [w423 w429 w431 w437] -> w419
          tunnel: [w422 w428 w430 w436] -> w418
          tunnel: [_ TRUE _ TRUE] -> w416
          frame #0 {
            n191 = Enqueue Element(queue=w426, element="Start" ("notification"), error in (no error)=w424) -> (queue out=w423:refnum<queue>, error out=w422:errorcluster)  [unwired: 1 in, 1 out]
          }
          frame #1 {
          }
          frame #2 {
            n192 = Enqueue Element(queue=w434, element="Stop" ("notification"), error in (no error)=w432) -> (queue out=w431:refnum<queue>, error out=w430:errorcluster)  [unwired: 1 in, 1 out]
          }
          frame #3 {
          }
        }
        n193 = event-data("Discard?"=w416) -> ()  [unwired: 1 in, 1 out]
      }
      event #4 {
        n194 = event-data() -> ()  [unwired: 2 out]
        n195 = local read "Square State"() -> (w441:T4)
        n196 = case shown="\"Start Wave\"" w441 {
          tunnel: w440 -> [w448 w453 w458 w461 w464]
          tunnel: w443 -> [w446 w451 w456 w460 w463]
          tunnel: [w445 w450 w455 w461 w464] -> w439
          tunnel: [w444 w449 w454 w460 w463] -> w442
          tunnel: [_ _ _ TRUE TRUE] -> w438
          frame #0 {
            n197 = Enqueue Element(queue=w448, element="Start" ("notification"), error in (no error)=w446) -> (queue out=w445:refnum<queue>, error out=w444:errorcluster)  [unwired: 1 in, 1 out]
          }
          frame #1 {
            n198 = Enqueue Element(queue=w453, element="Stop" ("notification"), error in (no error)=w451) -> (queue out=w450:refnum<queue>, error out=w449:errorcluster)  [unwired: 1 in, 1 out]
          }
          frame #2 {
            n199 = Enqueue Element(queue=w458, element="Stop" ("notification"), error in (no error)=w456) -> (queue out=w455:refnum<queue>, error out=w454:errorcluster)  [unwired: 1 in, 1 out]
          }
          frame #3 {
          }
          frame #4 {
          }
        }
        n200 = event-data("Discard?"=w438) -> ()  [unwired: 1 in, 1 out]
      }
      event #5 {
        n201 = event-data() -> ()  [unwired: 2 out]
        n202 = local read "Set Control"() -> (w473:cluster{"Set":bool, "Actuator Controls":T1})
        n203 = Unbundle By Name(w473) -> ("Actuator Controls"=w466:T1)
        n204 = local read "Square Control"() -> (w467:T5)
        n205 = local read "Ramp Control"() -> (w469:T2)
        n206 = Bundle By Name(cluster=w469, "Actuator Controls"=w466) -> (w468:T2)
        n207 = Bundle By Name(cluster=w467, "Actuator Controls"=w466) -> (w465:T5)
        n208 = call "Actuator Controls 2 Array.vi"("Actuator Controls"=w466) -> ("Array"=w470:dbl[])  [unwired: 10 in]
        n209 = local write "Control Voltage"(w470) -> ()
        n210 = local write "Square Control"(w465) -> ()
        n211 = local write "Ramp Control"(w468) -> ()
      }
      event #6 {
        n212 = event-data() -> ()  [unwired: 2 out]
        n213 = property on="Readings" class="WFChart (strict)"(error in=w475, "History Data"=T21 []) -> ()  [unwired: 1 in, 2 out]
      }
      event #7 {
        n214 = event-data() -> ("NewVal"=w486:i32, "OldVal"=w485:i32)  [unwired: 1 out]
        n215 = property on="Readings" class="WFChart (strict)"(error in=w483, "Active Plot"=w485) -> (error out=w484:errorcluster)  [unwired: 1 in, 1 out]
        n216 = property on="Readings" class="WFChart (strict)"(error in=w484, "Plot.Line Width"=u8 0) -> (error out=w481:errorcluster)  [unwired: 1 in, 1 out]
        n217 = property on="Readings" class="WFChart (strict)"(error in=w481, "Active Plot"=w486) -> (error out=w480:errorcluster)  [unwired: 1 in, 1 out]
        n218 = property on="Readings" class="WFChart (strict)"(error in=w480, "Plot.Line Width"=u8 3) -> (error out=w479:errorcluster)  [unwired: 1 in, 1 out]
      }
      event #8 {
        n219 = event-data() -> ()  [unwired: 2 out]
        n220 = property on="Readings" class="WFChart (strict)"(error in=w504) -> (error out=w503:errorcluster, "History Data"=w493:T21)  [unwired: 1 in, 1 out]
        n221 = for {
          tunnel: [w508] -> w506 mode=indexing
          tunnel: w493 -> [w507] mode=indexing
          n222 = Cluster To Array(cluster=w507) -> (array=w508:dbl[])
        }
        n223 = local read "Actuator"() -> (w491:i32)
        n224 = Index Array(array=w506, index (col)=w491) -> (element=w492:dbl[])  [unwired: 1 in]
        n225 = Array Max & Min(array=w492) -> (max value=w497:dbl, min value=w496:dbl)  [unwired: 2 out]
        n226 = Subtract(x=w497, y=w496) -> (x-y=w490:dbl)
        n227 = local read "Zoom Type"() -> (w500:T12)
        n228 = Multiply(x=w490, y=0.02) -> (x*y=w498:dbl)
        n229 = Absolute Value(x=w498) -> (abs(x)=w489:dbl)
        n230 = case shown="\"Lower Half\"" w500 {
          tunnel: w489 -> [w510 w518 w526 w535 w542]
          tunnel: w497 -> [w513 w519 w527 w531 w544]
          tunnel: w496 -> [w511 w521 w529 w532 w539]
          tunnel: [w512 w517 w525 w536 w543] -> w495
          tunnel: [w509 w520 w528 w537 w545] -> w494
          tunnel: w490 -> [_ w516 w524 w533 w541]
          tunnel: 0.98 ("y") -> [_ _ w522 _ w538]
          tunnel: 0.5 ("y") -> [_ w514 _ w530 _]
          frame #0 {
            n231 = Add(x=w513, y=w510) -> (x+y=w512:dbl)
            n232 = Subtract(x=w511, y=w510) -> (x-y=w509:dbl)
          }
          frame #1 {
            n233 = Multiply(x=w516, y=w514) -> (x*y=w515:dbl)
            n234 = Add(x=w519, y=w518) -> (x+y=w517:dbl)
            n235 = Add(x=w515, y=w521) -> (x+y=w520:dbl)
          }
          frame #2 {
            n236 = Multiply(x=w524, y=w522) -> (x*y=w523:dbl)
            n237 = Add(x=w527, y=w526) -> (x+y=w525:dbl)
            n238 = Add(x=w523, y=w529) -> (x+y=w528:dbl)
          }
          frame #3 {
            n239 = Multiply(x=w533, y=w530) -> (x*y=w534:dbl)
            n240 = Subtract(x=w532, y=w535) -> (x-y=w537:dbl)
            n241 = Subtract(x=w531, y=w534) -> (x-y=w536:dbl)
          }
          frame #4 {
            n242 = Multiply(x=w541, y=w538) -> (x*y=w540:dbl)
            n243 = Subtract(x=w539, y=w542) -> (x-y=w545:dbl)
            n244 = Subtract(x=w544, y=w540) -> (x-y=w543:dbl)
          }
        }
        n245 = property on="Readings" class="WFChart (strict)"(error in=w503, "YScale.Maximum"=w495) -> (error out=w502:errorcluster)  [unwired: 1 in, 1 out]
        n246 = property on="Readings" class="WFChart (strict)"(error in=w502, "YScale.Minimum"=w494) -> (error out=w501:errorcluster)  [unwired: 1 in, 1 out]
      }
      event #9 {
        n247 = event-data() -> ()  [unwired: 3 out]
        n248 = property on="Readings" class="WFChart (strict)"(error in=w548, "YScale.ScaleFit"=u8 1 ("Y Scale.Scale Fit")) -> (error out=w547:errorcluster)  [unwired: 1 in, 1 out]
      }
    }
    n249 = local read "Quit"() -> (w375:bool)
    n250 = Not(x=w375) -> (.not. x?=w370:bool)
  }
  n251 = while {
    shift-right: [w556] -> _
    shift-left: w29 -> [w562]
    shift-right: [w557] -> _
    shift-left: w22 -> [w561]
    tunnel: [w550] -> w28
    stop <- w550 stop-if-true
    n252 = Get Queue Status(queue=w562, error in (no error)=w561) -> (queue out=w559:refnum<queue>, error out=w558:errorcluster, # elements in queue=w560:i32)  [unwired: 1 in, 5 out]
    n253 = Wait (ms)(milliseconds to wait=u32 2000) -> ()  [unwired: 1 out]
    n254 = Greater Than 0?(x=w560) -> (x > 0?=w552:bool)
    n255 = And(x=w552, y="Logging") -> (x .and. y?=w553:T15)
    n256 = case shown="False" w553 {
      tunnel: w559 -> [w564 w572]
      tunnel: w558 -> [w563 w571]
      tunnel: [w563 w570] -> w557
      tunnel: [w564 w568] -> w556
      frame #0 {
      }
      frame #1 {
        n257 = Flush Queue(queue=w572, error in (no error)=w571) -> (queue out=w568:refnum<queue>, remaining elements=w569:cluster{dbl[]}[], error out=w567:errorcluster)
        n258 = for {
          tunnel: w569 -> [w587] mode=indexing
          shift-right: [w584] -> w566
          shift-left: "" -> [w583]
          n259 = Unbundle(w587) -> (w586:dbl[])
          n260 = call "Data 2 Record.vi"("Data"=w586) -> ("Records"=w585:string)  [unwired: 10 in]
          n261 = Concatenate Strings(w583, w585) -> (w584:string)
        }
        n262 = Open/Create/Replace File(file path (use dialog)="Log File Path", error in=w567, operation (0:open)=T22."open or create", access (0:read/write)=enum16{"read/write", "read-only", "write-only"}."write-only") -> (refnum out=w578:refnum<file>, error out=w577:errorcluster)  [unwired: 3 out]
        n263 = Set File Position(refnum=w578, from (0:start)=enum16{"start", "end", "current"}."end", error in=w577) -> (refnum out=w575:refnum<file>, error out=w576:errorcluster)  [unwired: 1 out]
        n264 = Write to Text File(file (use dialog)=w575, text=w566, error in=w576) -> (refnum out=w580:refnum<file>, error out=w581:errorcluster)  [unwired: 2 out]
        n265 = Close File(refnum=w580, error in=w581) -> (error out=w570:errorcluster)  [unwired: 1 out]
      }
    }
    n266 = local read "Quit"() -> (w555:bool)
    n267 = Not(x=w555) -> (.not. x?=w550:bool)
  }
  n268 = while "Display Loop" {
    shift-right: [w588] -> w36
    shift-left: w22 -> [w603]
    tunnel: [w590] -> w40
    shift-right: [w597] -> _
    shift-left: w29 -> [w598]
    stop <- w590 stop-if-true
    w605 = 6
    n269 = local read "Control Voltage"() -> (→"Command Voltage":dbl[])
    n270 = Wait Until Next ms Multiple(millisecond multiple=4) -> ()  [unwired: 1 out]
    n271 = call "DAQ Finite Read Servo Errors.vi"("error in"=w603, "Action"=DAQ_Read_Actions."Read") -> ("error out"=w602:errorcluster, "Average"=w599:dbl[])  [unwired: 3 in, 5 out]
    n272 = call <vilib>:"Clear Errors.vi"("error in (no error)"=w602) -> ("error out"=w600:errorcluster)  [unwired: 6 out]
    n273 = Delete From Array(array=w599, length=w605, index=0) -> (deleted portion=w595:dbl[], array with subset deleted=w606:dbl[])
    "LVDT Reading" <- w595
    n274 = Delete From Array(array=w606, length=w605, index=w605) -> (deleted portion=w593:dbl[], array with subset deleted=w594:dbl[])
    "Load Cell \nReading" <- w594
    "Servo Error Reading" <- w593
    n275 = local read "Readings"() -> (w596:T13)
    n276 = Enqueue Element(queue=w598, element=w599, error in (no error)=w600) -> (queue out=w597:refnum<queue>, error out=w588:errorcluster)  [unwired: 1 in, 1 out]
    n277 = case shown="\"LVDT\"" w596 {
      tunnel: w595 -> [w609 _ _]
      tunnel: w594 -> [_ w610 _]
      tunnel: w593 -> [_ _ w611]
      tunnel: [w609 w610 w611] -> w592
      frame #0 {
      }
      frame #1 {
      }
      frame #2 {
      }
    }
    n278 = local read "Quit"() -> (w607:bool)
    n279 = Not(x=w607) -> (.not. x?=w590:bool)
    n280 = local write "Write error out"(w588) -> ()
    n281 = Array To Cluster(array=w592) -> (cluster=→"Readings":T14)
  }
  n282 = Compound Arithmetic op=AND(w28, w40, w42, w38, w31, w9, w5) -> (w41:bool)
  n283 = call "DAQ Finite Read Servo Errors.vi"("error in"=w36, "Action"=DAQ_Read_Actions."Stop") -> ("error out"=→"Write error out":errorcluster)  [unwired: 3 in, 6 out]
  n284 = Not(x=w41) -> (.not. x?=w39:bool)
  n285 = flat-sequence {
    tunnel: w39 -> [w613]
    frame #0 {
      n286 = control-ref of="This VI"() -> (w612:refnum<vi>)
      n287 = local write "Quit"(w613) -> ()
      n288 = disable-structure shown="Disabled" {
        disable-tunnel: w612 -> [w614 _]
        frame #0 {
          n289 = invoke class="VI" method="FP.Close"(reference=w614) -> ()  [unwired: 2 in, 3 out]
        }
        frame #1 {
        }
      }
    }
  }
